vi "2.2、2.3、2.4.vi"() -> ()   [LabVIEW 2017]
panel:
  out "y":dbl
  in  "b":dbl
  in  "k":dbl
  in  "x":dbl
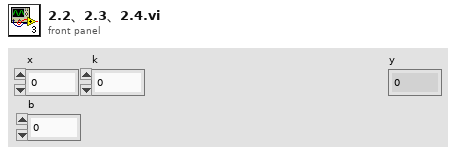
[diagram p1: front panel]
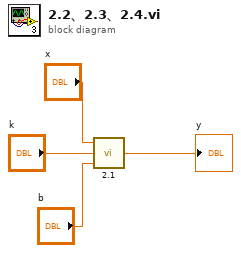
[diagram p0: block diagram]
diagram:
  n1 = call "2.1.vi"("b"="b", "k"="k", "x"="x") -> ("y"=→"y":dbl)
